vi "Configure Session.vi"(8 "error in":errorcluster, 11 "Plugin in":refnum<class "RPM Plugin.lvclass">) -> (0 "error out":errorcluster, 3 "Plugin out":refnum<class "RPM Plugin.lvclass">)   [LabVIEW 2020, in "RPM Plugin.lvlib" / "RPM Plugin.lvclass"]
uses:
  RPM Plugin.lvclass
  C:/Program Files/National Instruments/LabVIEW 2020/vi.lib/FlexLogger/SDK/PluginSDK.lvlibp/PEFClasses/SDK/Plugin/Plugin.lvclass
  RPM Plugin.lvclass/RPM Plugin.ctl
  <vilib>/FlexLogger/SDK/PluginSDK.lvlibp/PEFClasses/SDK/Channel/ParameterAccess/Read DBL.vi
  <vilib>/FlexLogger/SDK/PluginSDK.lvlibp/PEFClasses/SDK/Plugin/ParameterAccess/Read String.vi
  <vilib>/FlexLogger/SDK/PluginSDK.lvlibp/PEFClasses/SDK/Plugin/ParameterAccess/Read DBL.vi
  <vilib>/DAQmx/create/channels.llb/DAQmx Create Channel (CI-Frequency).vi
  <vilib>/FlexLogger/SDK/PluginSDK.lvlibp/PEFClasses/SDK/Plugin/Plugin.lvclass
  <vilib>/FlexLogger/SDK/PluginSDK.lvlibp/PEFClasses/SDK/Channel/Channel.lvclass
  C:/Program Files/National Instruments/LabVIEW 2020/vi.lib/FlexLogger/SDK/PluginSDK.lvlibp/PEFClasses/SDK/Processing Element/Processing Element.lvclass
  D:/AE/Transportation/Schwing Stetter/RPM Plugin/RPM Plugin Source Code/RPM Plugin.lvclass
  <resource>/objmgr/daqmx.rc
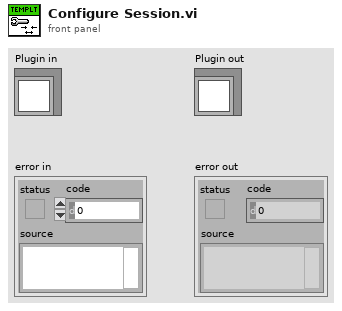
[diagram p1: front panel]
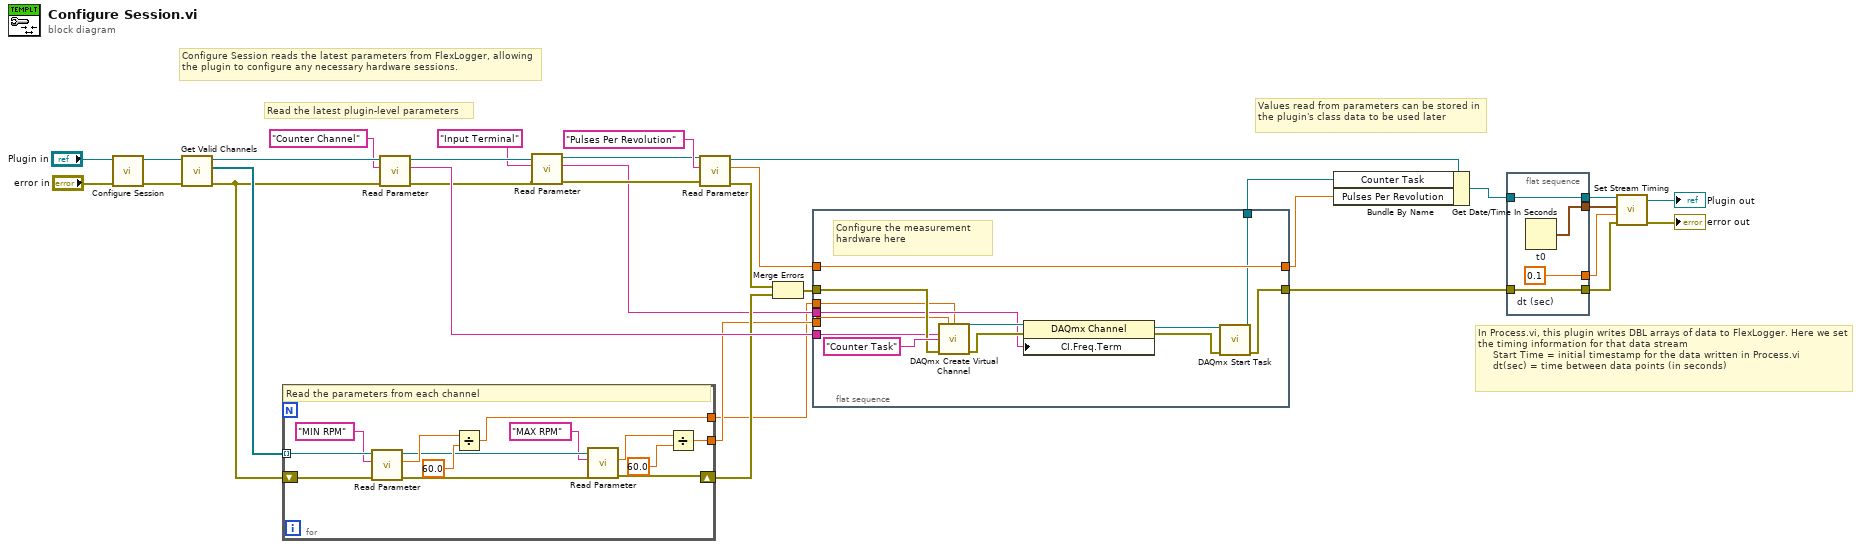
[diagram p0: block diagram]
diagram:
  # "Read the latest plugin-level parameters"
  # "Configure Session reads the latest parameters from FlexLogger, allowing the plugin to configure any necessary hardware sessions."
  # "Values read from parameters can be stored in the plugin's class data to be used later"
  # "In Process.vi, this plugin writes DBL arrays of data to FlexLogger. Here we set the timing information for that data stream\n     Start Time = initial timestamp for the data written in Process.vi\n     dt(sec) = time between data points (in seconds)"
  n1 = call-parent "Configure Session.vi"("error in (no error)"="error in", "Processing Element in"="Plugin in") -> ("error out"=w25:errorcluster, "Processing Element out"=w26:refnum<class "RPM Plugin.lvclass">)  [unwired: 8 in]
  n2 = call <vilib>:"Get Valid Channels.vi"("error in (no error)"=w25, "Plugin in"=w26) -> ("error out"=w13:errorcluster, "Channels"=w31:refnum<class "Channel.lvclass">[], "Plugin out"=w30:refnum<class "RPM Plugin.lvclass">)  [unwired: 7 in]
  n3 = for {
    tunnel: w31 -> [w46] mode=indexing
    tunnel: [w34] -> w4
    shift-right: [w36] -> w16
    shift-left: w13 -> [w44]
    tunnel: [w35] -> w3
    # "Read the parameters from each channel"
    n4 = call-poly <vilib>:"Read Parameter.vi"("error in (no error)"=w44, "Name"="MIN RPM", "Channel in"=w46) -> ("error out"=w40:errorcluster, "Value"=w43:dbl, "Channel out"=w41:refnum<class "Channel.lvclass">)  [unwired: 5 in, 1 out]
    n5 = Divide(x=w43, y=60.0) -> (x/y=w35:dbl)
    n6 = call-poly <vilib>:"Read Parameter.vi"("error in (no error)"=w40, "Name"="MAX RPM", "Channel in"=w41) -> ("error out"=w36:errorcluster, "Value"=w38:dbl)  [unwired: 5 in, 2 out]
    n7 = Divide(x=w38, y=60.0) -> (x/y=w34:dbl)
  }
  n8 = call-poly <vilib>:"Read Parameter.vi"("error in (no error)"=w13, "Name"="Counter Channel", "Plugin in"=w30) -> ("error out"=w8:errorcluster, "Value"=w23:string, "Plugin out"=w10:refnum<class "RPM Plugin.lvclass">)  [unwired: 5 in, 1 out]
  n9 = call-poly <vilib>:"Read Parameter.vi"("error in (no error)"=w8, "Name"="Input Terminal", "Plugin in"=w10) -> ("error out"=w7:errorcluster, "Value"=w5:string, "Plugin out"=w9:refnum<class "RPM Plugin.lvclass">)  [unwired: 5 in, 1 out]
  n10 = call-poly <vilib>:"Read Parameter.vi"("error in (no error)"=w7, "Name"="Pulses Per Revolution", "Plugin in"=w9) -> ("error out"=w15:errorcluster, "Value"=w24:dbl, "Plugin out"=w28:refnum<class "RPM Plugin.lvclass">)  [unwired: 5 in, 1 out]
  n11 = Merge Errors(w15, w16) -> (w14:errorcluster)
  n12 = flat-sequence {
    tunnel: [w48] -> w21
    tunnel: w14 -> [w53]
    tunnel: w24 -> [w59]
    tunnel: w23 -> [w51]
    tunnel: [w59] -> w2
    tunnel: w5 -> [w52]
    tunnel: w4 -> [w50]
    tunnel: w3 -> [w49]
    tunnel: [w47] -> w1
    frame #0 {
      # "Configure the measurement hardware here"
      n13 = call-poly <vilib>:"DAQmx Create Virtual Channel.vi"("maximum value"=w50, "minimum value"=w49, "counter"=w51, "name to assign"="Counter Task", "error in"=w53) -> ("task out"=w57:refnum<k21>, "error out"=w56:errorcluster)  [unwired: 9 in]
      n14 = property class="DAQmx Channel"(reference=w57, error in=w56, "CI.Freq.Term"=w52) -> (reference out=w55:refnum<k21>, error out=w54:errorcluster)
      n15 = call <vilib>:"DAQmx Start Task.vi"("task/channels in"=w55, "error in"=w54) -> ("task out"=w47:refnum<k21>, "error out"=w48:errorcluster)  [unwired: 12 in]
    }
  }
  n16 = Bundle By Name(cluster=w28, "Counter Task"=w1, "Pulses Per Revolution"=w2) -> (w22:refnum<class "RPM Plugin.lvclass">)
  n17 = flat-sequence {
    tunnel: [w63] -> w19
    tunnel: [w62] -> w17
    tunnel: w21 -> [w61]
    tunnel: [w61] -> w18
    tunnel: w22 -> [w60]
    tunnel: [w60] -> w20
    frame #0 {
      w62 = 0.1  # dt (sec)
      n18 = Get Date/Time In Seconds "t0"() -> (seconds since 1Jan1904=w63:timestamp)
    }
  }
  n19 = call-dynamic "Set Stream Timing.vi"("error in (no error)"=w18, "dt(sec)"=w17, "Start Time"=w19, "Plugin in"=w20) -> ("error out"=→"error out":errorcluster, "Plugin out"=→"Plugin out":refnum<class "RPM Plugin.lvclass">)  [unwired: 6 in]
